vi "Memory.Pointer.Move.vi"   [LabVIEW 2016, in "Memory Manager.lvlib" / "Memory.Pointer.lvclass"]
uses:
  Memory.Pointer.lvclass
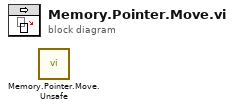
[diagram p0: block diagram]
diagram:
  n1 = call "Memory.Pointer.Move.Unsafe.vi"() -> ()  [unwired: 8 in, 4 out]
